vi "Alarm.vi"(3 "Lable":enum16{"UpDate", "loop", "delete", "clear"}(ring), 4 "Delete Row":i32, 6 "In":string[](array[string])) -> (1 "Out":string[][](array[string]))   [LabVIEW 2015]
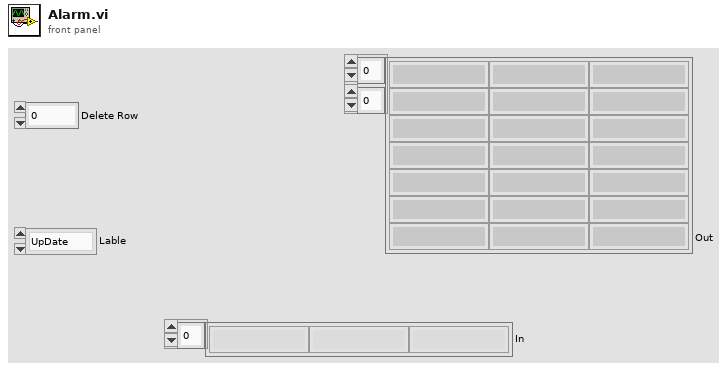
[diagram p1: front panel]
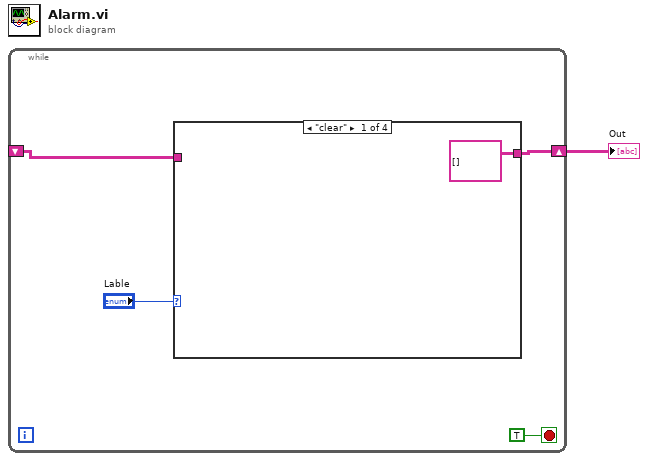
[diagram p0: block diagram]
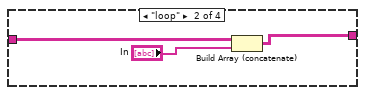
[diagram p2: hidden frame]
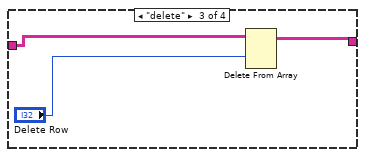
[diagram p3: hidden frame]
diagram:
  n1 = while {
    shift-right: [w4] -> w1
    shift-left: _ -> [w2]
    stop <- TRUE stop-if-true
    n2 = case shown="\"clear\"" "Lable" {
      tunnel: [string[][] [] w8 w10 w13] -> w4
      tunnel: w2 -> [_ w7 w11 w13]
      frame "clear" {
      }
      frame "loop" {
        n3 = Build Array (concatenate)(w7, "In") -> (w8:string[][])
      }
      frame "delete" {
        n4 = Delete From Array(array=w11, index (row)="Delete Row") -> (array with subset deleted=w10:string[][])  [unwired: 2 in, 1 out]
      }
      frame "UpDate" {
      }
    }
  }
  "Out" <- w1
